vi "getCamFrame.vi"(8 "error in (no error)":errorcluster, 11 "Cluster":T1) -> (0 "error out":errorcluster, 2 "Acquired Frames per Second":dbl, 3 "output cluster":T1)   [LabVIEW 2020]
doc: "Get last frame from a camera"
uses:
  controls/StateMachineVariables.ctl
  <vilib>/vision/Avi.llb/IMAQ AVI2 Refnum.ctl
  <vilib>/userDefined/High Color/IMAQdx.ctl
  <vilib>/vision/Deep Learning.llb/IMAQ DL Model Refnum.ctl
  <vilib>/vision/Image Controls.llb/IMAQ Image.ctl
  <vilib>/vision/driver/NI_Vision_Acquisition_Software.lvlib
  <vilib>/vision/NI_Vision_Development_Module.lvlib
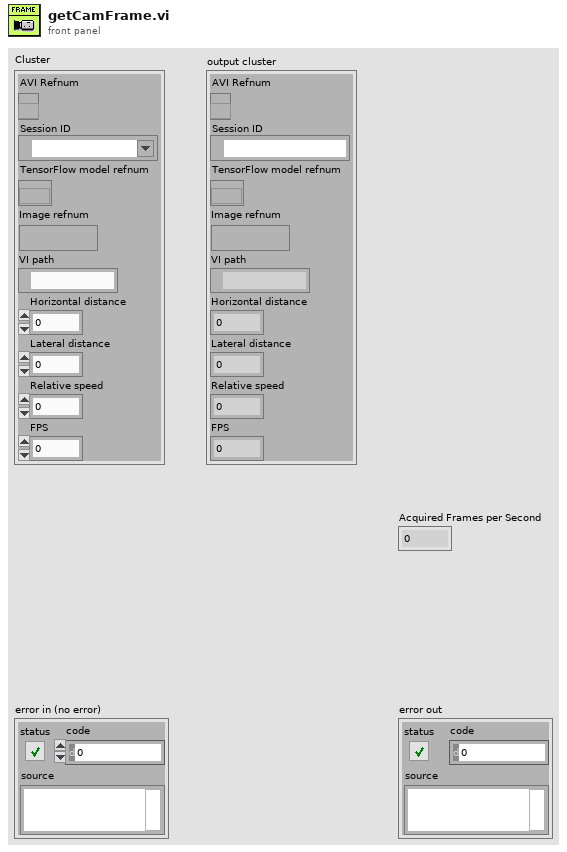
[diagram p1: front panel]
types:
  T1 = typedef "StateMachineVariables.ctl" = cluster{"AVI Refnum":T2, "Session ID":T3, "TensorFlow model refnum":T4, "Image refnum":T5, "VI path":path, "Horizontal distance":dbl, "Lateral distance":dbl, "Relative speed":dbl, "FPS":dbl}
  T2 = typedef "IMAQ AVI2 Refnum.ctl" = refnum<k20>
  T3 = typedef "IMAQdx.ctl" = refnum<k21>
  T4 = typedef "IMAQ DL Model Refnum.ctl" = refnum<k20>
  T5 = typedef "IMAQ Image.ctl" = refnum<image>
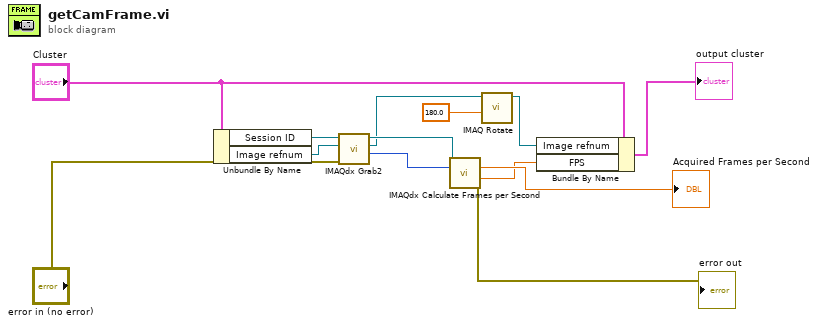
[diagram p0: block diagram]
diagram:
  n1 = Unbundle By Name("Cluster") -> ("Session ID"=w11:T3, "Image refnum"=w12:T5)
  n2 = call <vilib>:"IMAQdx Grab2.vi"("error in"="error in (no error)", "Image In"=w12, "Session In"=w11) -> ("Buffer Number Out"=w7:u32, "Image Out"=w1:T5, "Session Out"=w8:T3)  [unwired: 5 in, 1 out]
  n3 = call <vilib>:"IMAQdx Calculate Frames per Second.vi"("Session In"=w8, "Buffer Number"=w7) -> ("Acquired Frames per Second"=→"Acquired Frames per Second":dbl, "Processed Frames per Second"=w4:dbl, "error out"=→"error out":errorcluster)  [unwired: 7 in, 4 out]
  n4 = call "IMAQ Rotate"("Angle (degrees)"=sgl 180.0, "Image Src"=w1) -> ("Image Dst Out"=w2:T5)  [unwired: 8 in, 1 out]
  n5 = Bundle By Name(cluster="Cluster", "Image refnum"=w2, "FPS"=w4) -> (→"output cluster":T1)
